vi "add scan frequency(SubVI).vi"(10 "字符串":string) -> (0 "布尔 3":bool, 2 "连接的字符串":string)   [LabVIEW 2019, in "Add Seq.lvlib"]
uses:
  Add Seq.lvlib
panel:
  in  "cancel":bool
  in  "ok":bool
  in  "Frequency List(空格分隔)":string
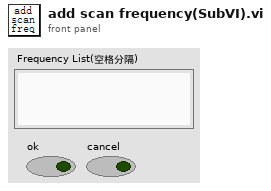
[diagram p1: front panel]
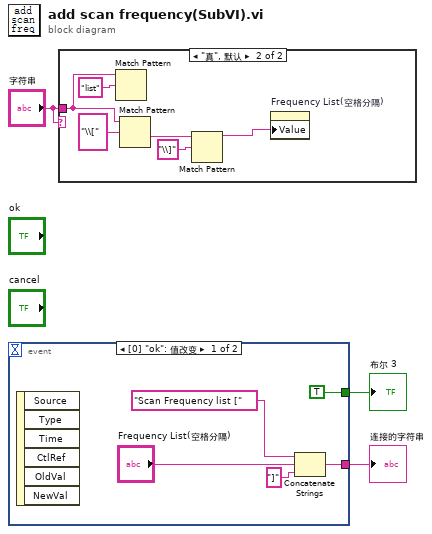
[diagram p0: block diagram]
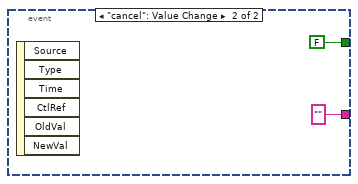
[diagram p3: hidden frame]
diagram:
  n1 = event shown="[0] \"ok\": 值改变" {
    selector: _ -> [_ _]
    dyn-events: _ -> [_ _]
    timeout: _ -> [_ _]
    tunnel: [TRUE FALSE] -> w3
    tunnel: [w4 ""] -> w1
    event "ok": Value Change {
      n2 = event-data() -> ()  [unwired: 1 in, 6 out]
      n3 = Concatenate Strings("Scan Frequency list [" ("字符串"), "Frequency List(空格分隔)", "]" ("字符串")) -> (w4:string)
    }
    event "cancel": Value Change {
      n4 = event-data() -> ()  [unwired: 1 in, 6 out]
    }
  }
  "布尔 3" <- w3
  "连接的字符串" <- w1
  n5 = case shown="\"真\", 默认" "字符串" {
    tunnel: "字符串" -> [_ w15]
    frame "" {
    }
    frame "真", Default {
      n6 = Match Pattern(string=w15, regular expression="list" ("正则表达式")) -> ()  [unwired: 1 in, 4 out]
      n7 = Match Pattern(string=w15, regular expression="\\[" ("正则表达式")) -> (after substring=w13:string)  [unwired: 1 in, 3 out]
      n8 = Match Pattern(string=w13, regular expression="\\]" ("正则表达式")) -> (before substring=w11:string)  [unwired: 1 in, 3 out]
      n9 = property on="Frequency List(空格分隔)" class="Str"("Value"=w11) -> ()  [unwired: 2 in, 2 out]
    }
  }
